vi "Sync Instrument UI.vi"() -> ()   [LabVIEW 2025, in "Synchronization.lvlib" / "Synchronization Instrument.lvclass"]
doc: "Copyright 2017 National Instruments Corporation\n\nLicensed under the Apache License, Version 2.0 (the \"License\"); you may not use this file except in compliance with the License. You may obtain a copy of the License at http://www.apache.org/licenses/LICENSE-2.0\nUnless required by applicable law or agreed to in writing, software distributed under the License is distributed on an \"AS IS\" BASIS, WITHOUT WARRANTIES OR CONDITIONS OF ANY KIND, either express or implied. See the License for the specific language governing permissions and limitations under the License."
uses:
  Synchronization Instrument.lvclass
  Users/Public/Documents/Sandia National Labs/TSS Plugin/CEF.lvlibp/Node/NodeRef.ctl
  Users/Public/Documents/Sandia National Labs/TSS Plugin/CEF.lvlibp/Node/CEF_Node.lvclass
  Users/Public/Documents/Sandia National Labs/TSS Plugin/CEF.lvlibp/Node/mainQref.ctl
  Users/Public/Documents/Sandia National Labs/TSS Plugin/CEF.lvlibp/Node/UserEventRef.ctl
  Users/Public/Documents/Sandia National Labs/TSS Plugin/Abstract Engine.lvlibp/Instrument configuration/Default Instrument.ctl
  Synchronization configuration/Sync Instrument Setting.ctl
  C:/Users/Public/Documents/Sandia National Labs/TSS Plugin/CEF.lvlibp/Node/CEF_Node.lvclass
  Synchronization Instrument.lvclass/Synchronization Instrument.ctl
  Synchronization configuration/Synchronization configuration.lvclass/Synchronization configuration.ctl
  Synchronization configuration/Read Sync Instrument Setting.vi
  Synchronization configuration/Write Sync Instrument Setting.vi
  <vilib>/Utility/error.llb/Trim Whitespace One-Sided.vi
  Synchronization configuration/Synchronization configuration.lvclass
  C:/Users/Public/Documents/Sandia National Labs/TSS Plugin/Abstract Engine.lvlibp/Instrument configuration/Instrument configuration.lvclass
  Users/Public/Documents/Sandia National Labs/TSS Plugin/Abstract Engine.lvlibp/Instrument configuration/Read Instrument Setting.vi
  Users/Public/Documents/Sandia National Labs/TSS Plugin/Abstract Engine.lvlibp/Instrument configuration/Write Instrument Setting.vi
  Users/Public/Documents/Sandia National Labs/TSS Plugin/Abstract Engine.lvlibp/Instrument configuration/Instrument configuration.lvclass
panel:
  in  "Sync":cluster{"Default":T1, "Setting":T2}={"Default"={"Type"="None", "Address"="None", "SW Alias"="None", "Description"="* Type = Class", "Enabled"=TRUE}, "Setting"={"Synchronization Clock"="Oscillator", "DDS Clock"=10000000.0, "SyncDivide1"="512", "SyncDivide2"="256"}} {"Setting"."DDS Clock" format="%#_6p"}
  in  "user event":T3
  in  "main queue":T4
  in  "node ref":T5
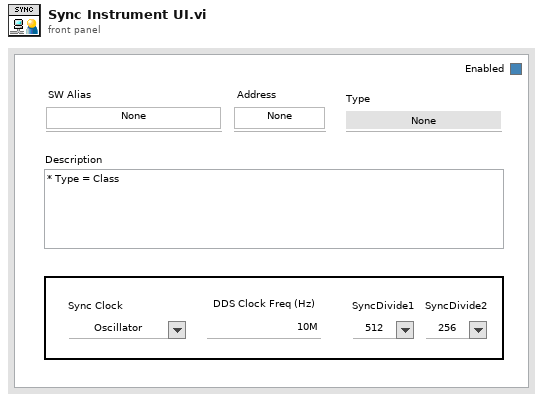
[diagram p1: front panel]
types:
  T1 = typedef "Abstract Engine.lvlibp/Instrument configuration.lvclass/Default Instrument.ctl" = cluster{"Type":string, "Address":string, "SW Alias":string, "Description":string, "Enabled":bool}
  T2 = typedef "Synchronization.lvlib/Synchronization configuration.lvclass/Sync Instrument Setting.ctl" = cluster{"Synchronization Clock":string, "DDS Clock":dbl, "SyncDivide1":string, "SyncDivide2":string}
  T3 = typedef "CEF.lvlibp/CEF_Node.lvclass/UserEventRef.ctl" = refnum<user-event>
  T4 = typedef "CEF.lvlibp/CEF_Node.lvclass/mainQref.ctl" = refnum<queue>
  T5 = typedef "CEF.lvlibp/CEF_Node.lvclass/NodeRef.ctl" = refnum<data-value>
  T6 = cluster{"Instrument Setting":T1, "Sync Instrument Setting":T2}
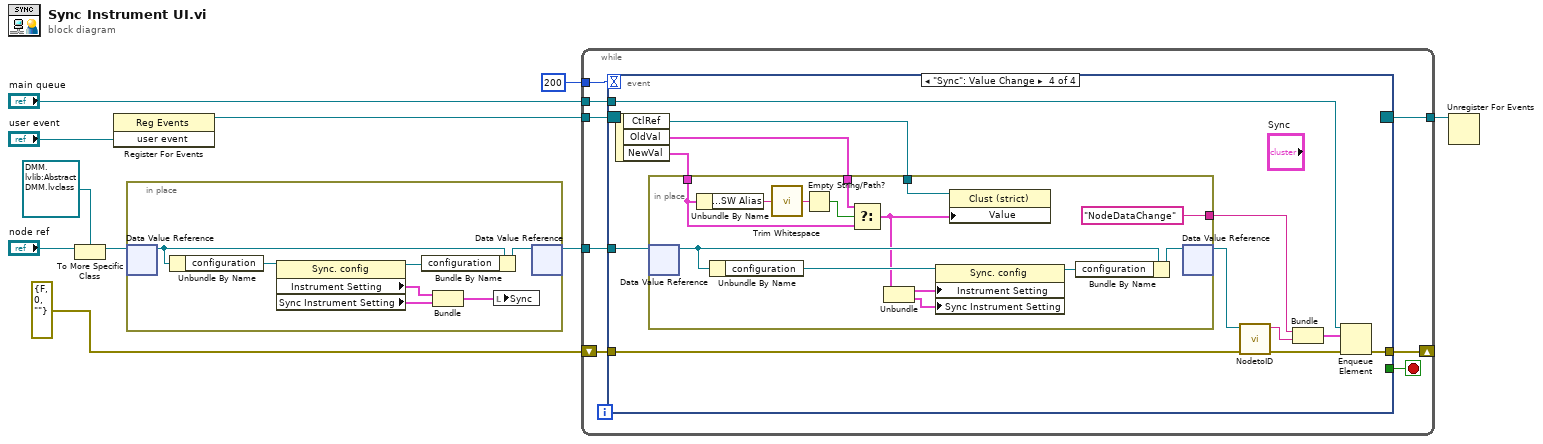
[diagram p0: block diagram]
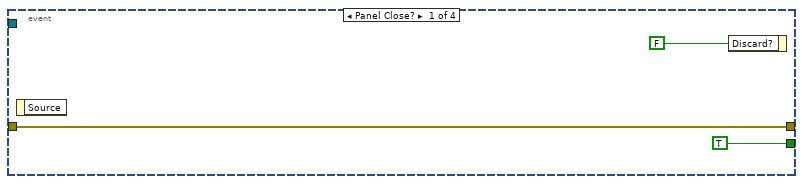
[diagram p2: hidden frame]
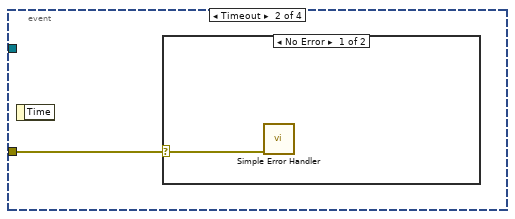
[diagram p3: hidden frame]
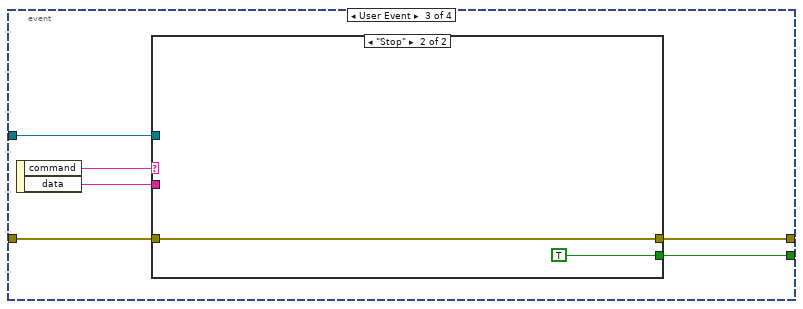
[diagram p5: hidden frame]
diagram:
  n1 = To More Specific Class(target class=refnum<data-value> refnum ("data value reference"), reference="node ref") -> (specific class reference=w8:refnum<data-value>)  [unwired: 1 in, 1 out]
  n2 = register-events("user event") -> (reference out=w10:refnum<event-registration>)  [unwired: 2 in, 1 out]
  n3 = in-place {
    # "Initialize the front panel controls when loaded"
    n4 = in-place-dvr #1(w8) -> (w15:refnum<class "Synchronization Instrument.lvclass">)  [unwired: 1 out]
    n5 = Unbundle By Name(w15) -> ("configuration"=w17:refnum<class "Synchronization configuration.lvclass">)
    n6 = property class="Sync. config"(reference=w17) -> (reference out=w14:refnum<class "Synchronization configuration.lvclass">, "Instrument Setting"=w11:T1, "Sync Instrument Setting"=w13:T2)  [unwired: 1 in, 1 out]
    n7 = Bundle By Name(cluster=w15, "configuration"=w14) -> (w16:refnum<class "Synchronization Instrument.lvclass">)
    n8 = Bundle("Instrument Setting"=w11, "Sync Instrument Setting"=w13) -> (w12:T6)  [unwired: 1 in]
    n9 = local write "Sync"(w12) -> ()
    n10 = in-place-dvr #1(w16) -> (w7:refnum<data-value>)  [unwired: 1 out]
  }
  n11 = while {
    tunnel: w7 -> [w25]
    tunnel: w10 -> [w24]
    tunnel: [w23] -> w9
    tunnel: 200 -> [w20]
    tunnel: "main queue" -> [w18]
    shift-right: [w19] -> _
    shift-left: errorcluster {"status"=FALSE, "code"=0, "source"=""} ("error out") -> [w21]
    stop <- w22 stop-if-true
    n12 = event shown="[3] \"Sync\": Value Change" {
      selector: w24 -> [_ _ _ _]
      dyn-events: [_ _ _ _] -> w23
      timeout: w20 -> [_ _ _ _]
      tunnel: w25 -> [_ _ w32 w50]
      tunnel: [TRUE _ w36 _] -> w22
      tunnel: [w27 _ w33 w51] -> w19
      tunnel: w21 -> [w27 w29 w34 w41]
      tunnel: w18 -> [_ _ _ w45]
      event Panel Close? {
        n13 = event-data() -> ()  [unwired: 1 in, 1 out]
        n14 = event-data("Discard?"=FALSE) -> ()  [unwired: 1 in, 1 out]
      }
      event Timeout {
        n15 = event-data() -> ()  [unwired: 1 in, 1 out]
        n16 = case shown="No Error" w29 {
          selector: w29 -> [w30 _]
          frame No Error {
            n17 = call <vilib>:"Simple Error Handler.vi"("error in (no error)"=w30) -> ()  [unwired: 4 in, 5 out]
          }
          frame Error {
          }
        }
      }
      event User Event {
        n18 = event-data() -> ("command"=w31:string, "data"=w35:string)  [unwired: 1 in]
        n19 = case shown="\"Stop\"" w31 {
          tunnel: [_ TRUE] -> w36
          tunnel: w35 -> [_ _]
          tunnel: w34 -> [w37 w38]
          tunnel: [w37 w38] -> w33
          tunnel: w32 -> [_ _]
          frame Default {
          }
          frame "Stop" {
          }
        }
      }
      event "Sync": Value Change {
        n20 = event-data() -> ("CtlRef"=w46:refnum<vi>, "OldVal"=w48:cluster{"Default":T1, "Setting":T2}, "NewVal"=w47:cluster{"Default":T1, "Setting":T2})  [unwired: 1 in]
        n21 = in-place {
          in-place-border: w48 -> [w61]
          in-place-border: w47 -> [w59]
          in-place-border: w46 -> [w57]
          in-place-border: ["NodeDataChange" ("Message Name")] -> w44
          n22 = in-place-dvr #2(w50) -> (w65:refnum<class "Synchronization Instrument.lvclass">)  [unwired: 1 out]
          n23 = Unbundle By Name(w59) -> ("Default.SW Alias"=w60:string)
          n24 = Unbundle By Name(w65) -> ("configuration"=w64:refnum<class "Synchronization configuration.lvclass">)
          n25 = call <vilib>:"Trim Whitespace.vi"("string"=w60) -> ("trimmed string"=w56:string)  [unwired: 1 in]
          n26 = Empty String/Path?(string/path=w56) -> (empty?=w58:bool)
          n27 = Select(t=w61, s=w58, f=w59) -> (s? t:f=w55:cluster{"Default":T1, "Setting":T2})
          n28 = Unbundle(w55) -> ("Default"=w54:T1, "Setting"=w53:T2)
          n29 = property class="Sync. config"(reference=w64, "Instrument Setting"=w54, "Sync Instrument Setting"=w53) -> (reference out=w62:refnum<class "Synchronization configuration.lvclass">)  [unwired: 1 in, 1 out]
          n30 = property class="Clust (strict)"(reference=w57, "Value"=w55) -> ()  [unwired: 1 in, 2 out]
          n31 = Bundle By Name(cluster=w65, "configuration"=w62) -> (w63:refnum<class "Synchronization Instrument.lvclass">)
          n32 = in-place-dvr #2(w63) -> (w49:refnum<data-value>)  [unwired: 1 out]
        }
        n33 = call "NodetoID.vi"("error in"=w41, "node ref"=w49) -> ("error out"=w40:errorcluster, "ID"=w43:string)  [unwired: 8 in]
        n34 = Bundle("Message Name"=w44, "ID"=w43) -> (w42:cluster{"Message Name":string, "ID":string})  [unwired: 1 in]
        n35 = Enqueue Element(queue=w45, element=w42, error in (no error)=w40) -> (error out=w51:errorcluster)  [unwired: 1 in, 2 out]
      }
    }
  }
  n36 = Unregister For Events(event registration refnum=w9) -> ()  [unwired: 1 in, 1 out]
